vi "Module Init.vi"(8 "error in (no error)":errorcluster, 11 "Historian Module in":refnum<class "Historian Module.lvclass">) -> (0 "error out":errorcluster, 3 "Historian Module out":refnum<class "Historian Module.lvclass">)   [LabVIEW 2020, in "VolatusHistorian.lvlib" / "Historian Module.lvclass"]
uses:
  Historian Module.lvclass
  C:/dev/lv20CE/relink/lv-volatus/Volatus/Module/Module.lvclass
  Volatus/Module/Module.lvclass/Module.ctl
  Volatus/MessageQ/MessageQ.lvclass/MessageQ.ctl
  Volatus/MessageQ/Send.vi
  Historian Module.lvclass/Historian Module.ctl
  Volatus/Module/Module.lvclass
  C:/dev/lv20CE/relink/lv-volatus/VolatusHistorian/Historian Module/Historian Module.lvclass
  History Data Controller/History Data Controller.lvclass
  Volatus/VolatusAPI/VolatusAPI.lvclass
  C:/dev/lv20CE/relink/lv-http-server/HTTP Server/Controller/Controller.lvclass
  C:/dev/lv20CE/relink/lv-http-server/HTTP Server/Handler/Handler.lvclass
  C:/dev/lv20CE/relink/lv-volatus/VolatusHistorian/History Data Controller/History Data Controller.lvclass
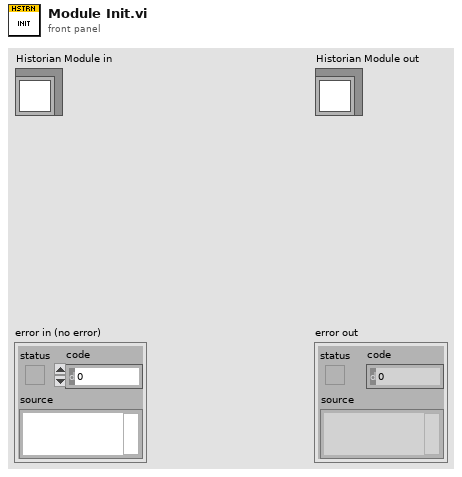
[diagram p1: front panel]
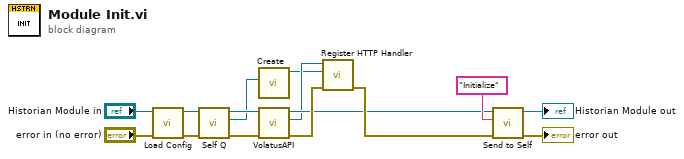
[diagram p0: block diagram]
diagram:
  n1 = call "Load Config.vi"("error in (no error)"="error in (no error)", "Historian Module in"="Historian Module in") -> ("error out"=w12:errorcluster, "Historian Module out"=w8:refnum<class "Historian Module.lvclass">)  [unwired: 8 in]
  n2 = call "Self Q.vi"("Module in"=w8) -> ("Self Q"=w4:refnum<class "MessageQ.lvclass">, "Module out"=w5:refnum<class "Historian Module.lvclass">)  [unwired: 9 in]
  n3 = call "Create.vi"("Historian MsgQ"=w4) -> ("History Data Controller out"=w1:refnum<class "History Data Controller.lvclass">)  [unwired: 9 in, 1 out]
  n4 = call "VolatusAPI.vi"("Module in"=w5) -> ("VolatusAPI"=w2:refnum<class "VolatusAPI.lvclass">, "Module out"=w3:refnum<class "Historian Module.lvclass">)  [unwired: 9 in]
  n5 = call "Register HTTP Handler.vi"("error in (no error)"=w12, "Handler"=w1, "VolatusAPI in"=w2) -> ("error out"=w13:errorcluster)  [unwired: 7 in, 1 out]
  n6 = call "Send to Self.vi"("error in (no error)"=w13, "Message ID"="Initialize", "Module in"=w3) -> ("error out"=→"error out":errorcluster, "Module out"=→"Historian Module out":refnum<class "Historian Module.lvclass">)  [unwired: 7 in]
